vi "set_params.vi"(8 "error in (no error)":errorcluster caption="entrée d'erreur (pas d'erreur)", 11 "SpectralClustering.lvclass 2":refnum<class "SpectralClustering.lvclass">) -> (0 "error out":errorcluster caption="sortie d'erreur", 3 "SpectralClustering.lvclass":refnum<class "SpectralClustering.lvclass">)   [LabVIEW 2020, in "SpectralClustering.lvclass"]
uses:
  SpectralClustering.lvclass
  SpectralClustering.lvclass/SpectralClustering.ctl
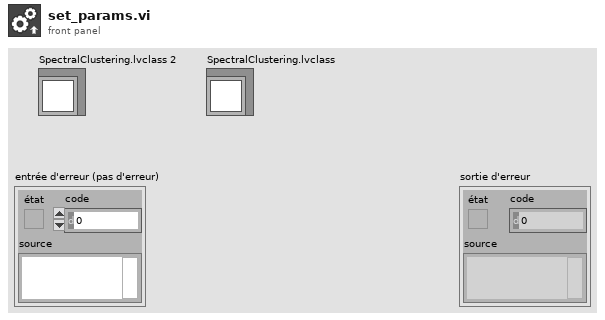
[diagram p1: front panel]
types:
  T1 = typedef "spectral_clustering_params.ctl" = cluster{"n_clusters":dbl, "eigen_solver":string, "n_components":cluster{"n_components_type":string, "n_components_int":dbl}, "random_state":dbl, "n_init":dbl, "gamma":dbl, "affinity":string, "n_neighbors":dbl, "eigen_tol":dbl, "assign_labels":string, "degree":dbl, "coef0":dbl, "n_jobs":dbl, "verbose":bool}
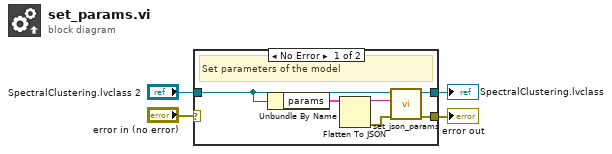
[diagram p0: block diagram]
diagram:
  n1 = case shown="No Error" "error in (no error)" {
    selector: "error in (no error)" -> [_ w12]
    tunnel: [w7 w12] -> w3
    tunnel: [w8 w11] -> w1
    tunnel: "SpectralClustering.lvclass 2" -> [w5 w11]
    frame No Error {
      # "Set parameters of the model"
      n2 = Unbundle By Name(w5) -> ("params"=w10:T1)
      n3 = Flatten To JSON(anything=w10) -> (JSON string=w9:string, 11:w6:errorcluster)  [unwired: 2 in]
      n4 = call-dynamic "set_json_params.vi"("error in (no error)"=w6, "params"=w9, "Model en entrée"=w5) -> ("error out"=w7:errorcluster, "Model en sortie"=w8:refnum<class "SpectralClustering.lvclass">)  [unwired: 7 in]
    }
    frame Error {
    }
  }
  "error out" <- w3
  "SpectralClustering.lvclass" <- w1
